vi "Wave2D_Cal U1.vi"(11 "Wave2D Data In":T1={"PDE"={"k"=0.0, "a"=0.0, "F(t, x, y)"=[]}, "Domain"={"t"={"initial t"=0.0, "final t"=0.0, "# of t-points"=0}, "x"={"start x"=0.0, "end x"=0.0, "# of x-points"=0}, "y"={"start y"=0.0, "end y"=0.0, "# of y-points"=11}, "delta"={"delta t"=0.0, "delta x"=0.0, "delta y"=0.0}}, "BC"={"Start X"={"type"=0, "Value"=[]}, "End X"={"type"=0, "Value"=[]}, "Start Y"={"type"=0, "Value"=[]}, "End Y"={"type"=0, "Value"=[]}}, "Corner"={"Start X & Start Y"=[], "Start X & End Y"=[], "End X & Start Y"=[], "End X & End Y"=[]}, "IC"={"Value"=[], "Derivative"=[]}, "P"={"Sub Diag"=[], "Diag"=[], "Super Diag"=[], "P"=[]}, "LU of P"={"L"=[], "U"={"Diag"=[], "Super Diag"=[], "2nd Super Diag"=[]}, "Pivot"=[]}, "Q"={"Sub Diag"=[], "Diag"=[], "Super Diag"=[], "Q"=[]}, "LU of Q"={"L"=[], "U"={"Diag"=[], "Super Diag"=[], "2nd Super Diag"=[]}, "Pivot"=[]}, "State"={"U"=[], "Old U"=[], "V&W"=[], "x start index"=0, "x length"=0, "y start index"=0, "y length"=0}} {"BC"."End Y"."type" items=["Dirichlet", "Neumann"]; "BC"."Start Y"."type" items=["Dirichlet", "Neumann"]; "BC"."End X"."type" items=["Dirichlet", "Neumann"]; "BC"."Start X"."type" items=["Dirichlet", "Neumann"]}) -> (3 "Wave2D Data Out":T1={"PDE"={"k"=0.0, "a"=0.0, "F(t, x, y)"=[]}, "Domain"={"t"={"initial t"=0.0, "final t"=0.0, "# of t-points"=0}, "x"={"start x"=0.0, "end x"=0.0, "# of x-points"=0}, "y"={"start y"=0.0, "end y"=0.0, "# of y-points"=11}, "delta"={"delta t"=0.0, "delta x"=0.0, "delta y"=0.0}}, "BC"={"Start X"={"type"=0, "Value"=[]}, "End X"={"type"=0, "Value"=[]}, "Start Y"={"type"=0, "Value"=[]}, "End Y"={"type"=0, "Value"=[]}}, "Corner"={"Start X & Start Y"=[], "Start X & End Y"=[], "End X & Start Y"=[], "End X & End Y"=[]}, "IC"={"Value"=[], "Derivative"=[]}, "P"={"Sub Diag"=[], "Diag"=[], "Super Diag"=[], "P"=[]}, "LU of P"={"L"=[], "U"={"Diag"=[], "Super Diag"=[], "2nd Super Diag"=[]}, "Pivot"=[]}, "Q"={"Sub Diag"=[], "Diag"=[], "Super Diag"=[], "Q"=[]}, "LU of Q"={"L"=[], "U"={"Diag"=[], "Super Diag"=[], "2nd Super Diag"=[]}, "Pivot"=[]}, "State"={"U"=[], "Old U"=[], "V&W"=[], "x start index"=0, "x length"=0, "y start index"=0, "y length"=0}} {"BC"."End Y"."type" items=["Dirichlet", "Neumann"]; "BC"."Start Y"."type" items=["Dirichlet", "Neumann"]; "BC"."End X"."type" items=["Dirichlet", "Neumann"]; "BC"."Start X"."type" items=["Dirichlet", "Neumann"]})   [LabVIEW 2020, in "NI_PDE.lvlib"]
uses:
  <vilib>/gmath/NI_PDE.lvlib
  <vilib>/gmath/pde.llb/Wave2D/Wave2D_Data.ctl
  <vilib>/gmath/pde.llb/Common/PDE_BC Type.ctl
  <vilib>/Analysis/Matrix/Datatypes/RealMatrix.ctl
  <vilib>/Analysis/Matrix/NI_Matrix.lvlib
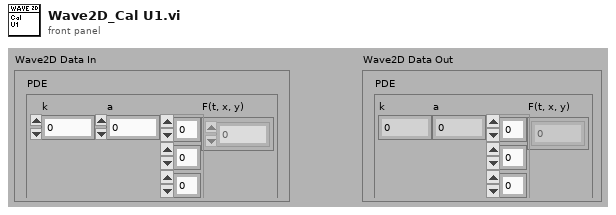
[diagram p1: front panel]
types:
  T1 = typedef "NI_PDE.lvlib/Wave2D_Data.ctl" = cluster{"PDE":cluster{"k":dbl, "a":dbl, "F(t, x, y)":dbl[][][]}, "Domain":cluster{"t":cluster{"initial t":dbl, "final t":dbl, "# of t-points":i32}, "x":cluster{"start x":dbl, "end x":dbl, "# of x-points":i32}, "y":cluster{"start y":dbl, "end y":dbl, "# of y-points":i32}, "delta":cluster{"delta t":dbl, "delta x":dbl, "delta y":dbl}}, "BC":cluster{"Start X":cluster{"type":T2, "Value":dbl[][]}, "End X":cluster{"type":T2, "Value":dbl[][]}, "Start Y":cluster{"type":T2, "Value":dbl[][]}, "End Y":cluster{"type":T2, "Value":dbl[][]}}, "Corner":cluster{"Start X & Start Y":dbl[], "Start X & End Y":dbl[], "End X & Start Y":dbl[], "End X & End Y":dbl[]}, "IC":cluster{"Value":dbl[][], "Derivative":dbl[][]}, "P":cluster{"Sub Diag":dbl[], "Diag":dbl[], "Super Diag":dbl[], "P":T3}, "LU of P":cluster{"L":dbl[], "U":cluster{"Diag":dbl[], "Super Diag":dbl[], "2nd Super Diag":dbl[]}, "Pivot":i32[]}, "Q":cluster{"Sub Diag":dbl[], "Diag":dbl[], "Super Diag":dbl[], "Q":T3}, "LU of Q":cluster{"L":dbl[], "U":cluster{"Diag":dbl[], "Super Diag":dbl[], "2nd Super Diag":dbl[]}, "Pivot":i32[]}, "State":cluster{"U":dbl[][], "Old U":dbl[][], "V&W":dbl[][], "x start index":i32, "x length":i32, "y start index":i32, "y length":i32}}
  T2 = typedef "NI_PDE.lvlib/PDE_BC Type.ctl" = i32
  T3 = typedef "NI_Matrix.lvlib/RealMatrix.ctl" = dbl[][]
  T4 = cluster{"Sub Diag":dbl[], "Diag":dbl[], "Super Diag":dbl[], "P":T3}
  T5 = cluster{"Sub Diag":dbl[], "Diag":dbl[], "Super Diag":dbl[], "Q":T3}
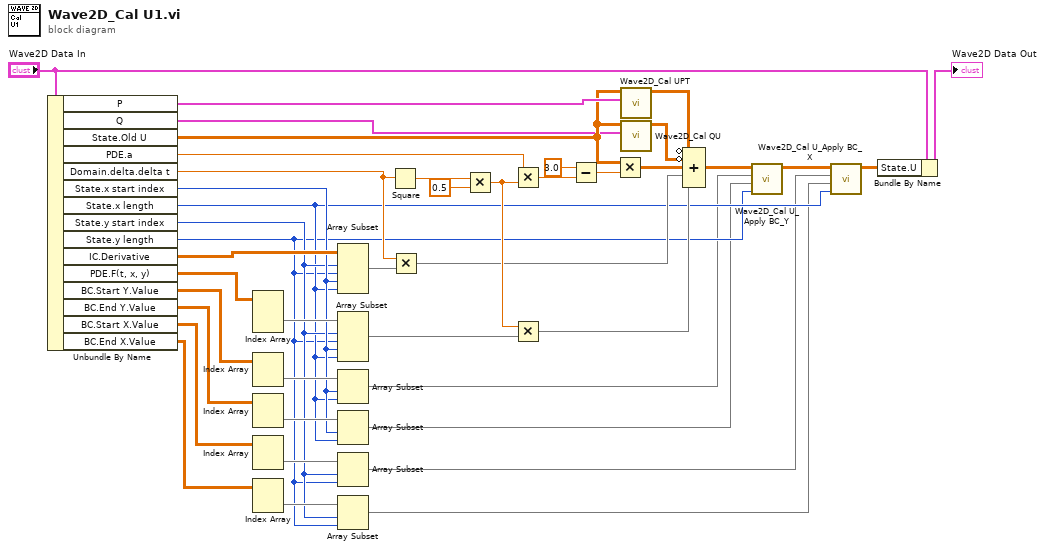
[diagram p0: block diagram]
diagram:
  n1 = Unbundle By Name("Wave2D Data In") -> ("P"=w10:T4, "Q"=w8:T5, "State.Old U"=w9:dbl[][], "PDE.a"=w37:dbl, "Domain.delta.delta t"=w31:dbl, "State.x start index"=w18:i32, "State.x length"=w7:i32, "State.y start index"=w11:i32, "State.y length"=w6:i32, "IC.Derivative"=w32:dbl[][], "PDE.F(t, x, y)"=w29:dbl[][][], "BC.Start Y.Value"=w17:dbl[][], "BC.End Y.Value"=w16:dbl[][], "BC.Start X.Value"=w13:dbl[][], "BC.End X.Value"=w12:dbl[][])
  n2 = Index Array(array=w29) -> (element=w28:dbl[][])  [unwired: 3 in]
  n3 = Index Array(array=w17) -> (element=w20:dbl[])  [unwired: 2 in]
  n4 = Index Array(array=w16) -> (element=w19:dbl[])  [unwired: 2 in]
  n5 = Index Array(array=w13) -> (element=w14:dbl[])  [unwired: 2 in]
  n6 = Index Array(array=w12) -> (element=w15:dbl[])  [unwired: 2 in]
  n7 = Array Subset(array=w32, index (row)=w11, length (row)=w6, index (col)=w18, length (col)=w7) -> (w30:dbl[][])
  n8 = Array Subset(array=w28, index (row)=w11, length (row)=w6, index (col)=w18, length (col)=w7) -> (w27:dbl[][])
  n9 = Array Subset(array=w20, index=w18, length=w7) -> (w4:dbl[])
  n10 = Array Subset(array=w19, index=w18, length=w7) -> (w3:dbl[])
  n11 = Array Subset(array=w14, index=w11, length=w6) -> (w2:dbl[])
  n12 = Array Subset(array=w15, index=w11, length=w6) -> (w1:dbl[])
  n13 = Square(x=w31) -> (x^2=w38:dbl)
  n14 = Multiply(x=w31, y=w30) -> (x*y=w25:dbl[][])
  n15 = Multiply(x=w38, y=0.5 ("value")) -> (x*y=w26:dbl)
  n16 = Multiply(x=w37, y=w26) -> (x*y=w40:dbl)
  n17 = Multiply(x=w26, y=w27) -> (x*y=w24:dbl[][])
  n18 = Subtract(x=3.0, y=w40) -> (x-y=w36:dbl)
  n19 = Multiply(x=w9, y=w36) -> (x*y=w35:dbl[][])
  n20 = call <vilib>:"Wave2D_Cal UPT.vi"("P"=w10, "U"=w9) -> ("UPT"=w33:dbl[][])  [unwired: 9 out]
  n21 = call <vilib>:"Wave2D_Cal QU.vi"("Q"=w8, "U"=w9) -> ("QU"=w34:dbl[][])  [unwired: 9 out]
  n22 = Compound Arithmetic op=ADD(invert w33, invert w34, w35, w25, w24) -> (w23:dbl[][])
  n23 = call <vilib>:"Wave2D_Cal U_Apply BC_Y.vi"("y length"=w6, "End Y Value"=w3, "Start Y Value"=w4, "U In"=w23) -> ("U Out"=w22:dbl[][])  [unwired: 2 in, 5 out]
  n24 = call <vilib>:"Wave2D_Cal U_Apply BC_X.vi"("x length"=w7, "End X Value"=w1, "Start X Value"=w2, "U In"=w22) -> ("U Out"=w21:dbl[][])  [unwired: 2 in, 5 out]
  n25 = Bundle By Name(cluster="Wave2D Data In", "State.U"=w21) -> (→"Wave2D Data Out":T1)
